vi "ErrorSum.vi"(10 "Smooth Vel":dbl[][](array[numeric]), 11 "Orig Vel":dbl[][](array[numeric])) -> (3 "Difference":dbl)   [LabVIEW 2016]
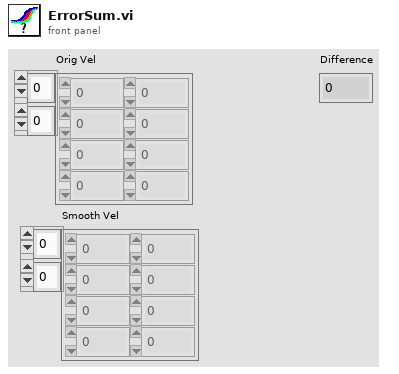
[diagram p1: front panel]
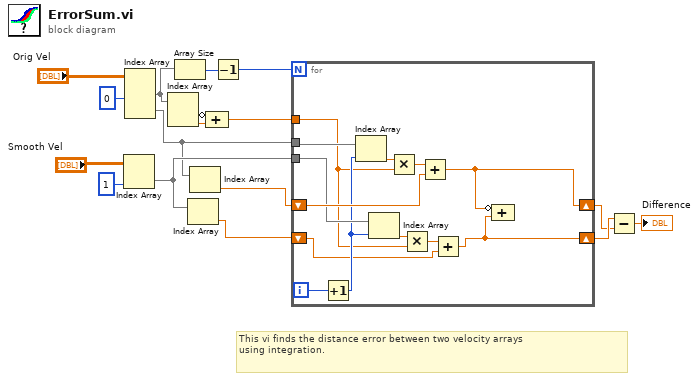
[diagram p0: block diagram]
diagram:
  # "This vi finds the distance error between two velocity arrays\nusing integration."
  n1 = Index Array(array="Smooth Vel", index (col)=1 ("disabled index (col)")) -> (element=w7:dbl[])  [unwired: 1 in]
  n2 = Index Array(array="Orig Vel", index (col) #1=0 ("disabled index (col)")) -> (element #1=w13:dbl[], element #2=w6:dbl[])  [unwired: 3 in]
  n3 = Index Array(array=w13) -> (element #1=w16:dbl, element #2=w15:dbl)  [unwired: 2 in]
  n4 = Array Size(array=w13) -> (size(s)=w12:i32)
  n5 = Index Array(array=w7) -> (element=w4:dbl)  [unwired: 1 in]
  n6 = Index Array(array=w6) -> (element=w5:dbl)  [unwired: 1 in]
  n7 = Compound Arithmetic op=ADD(invert w16, w15) -> (w10:dbl)
  n8 = Decrement(x=w12) -> (x-1=w11:i32)
  n9 = for {
    N: w11 -> [_]
    tunnel: w10 -> [w21]
    tunnel: w6 -> [w30]
    tunnel: w7 -> [w23]
    shift-right: [w18] -> w3
    shift-left: w4 -> [w20]
    shift-right: [w19] -> w2
    shift-left: w5 -> [w26]
    i -> [w29]
    n10 = Increment(x=w29) -> (x+1=w22:i32)
    n11 = Index Array(array=w30, index=w22) -> (element=w28:dbl)
    n12 = Index Array(array=w23, index=w22) -> (element=w24:dbl)
    n13 = Multiply(x=w28, y=w21) -> (x*y=w27:dbl)
    n14 = Multiply(x=w24, y=w21) -> (x*y=w25:dbl)
    n15 = Add(x=w27, y=w26) -> (x+y=w19:dbl)
    n16 = Add(x=w25, y=w20) -> (x+y=w18:dbl)
    n17 = Compound Arithmetic op=ADD(invert w19, w18) -> ()  [unwired: 1 out]
  }
  n18 = Subtract(x=w3, y=w2) -> (x-y=→"Difference":dbl)
